vi "Processing_data_subvi_V23.vi"() -> ()   [LabVIEW 2025]
uses:
  <vilib>/Analysis/3filter.llb/Filter Passband Type.ctl
  <vilib>/Analysis/baseanly.llb/Mean (DBL).vi
  <vilib>/Utility/file.llb/Read Delimited Spreadsheet (DBL).vi
  <vilib>/Analysis/1siggen.llb/Ramp Pattern by Delta.vi
  <vilib>/Analysis/3filter.llb/Butterworth Filter (DBL).vi
  <vilib>/addons/Time Series Analysis/Series Preprocess.llb/TSA Moving Average (Array).vi
  <vilib>/addons/Time Series Analysis/Correlation and Spectral Analysis.llb/TSA AR Spectrum (Array).vi
  <vilib>/Analysis/NI_AAL_SigProc.lvlib
  <vilib>/Analysis/NI_AALBase.lvlib
  <vilib>/Analysis/NI_AALPro.lvlib
  <vilib>/addons/_Advanced Signal Processing/NI_AdvSigProcTSA.lvlib
panel:
  in  "Path":path
  out "TABLE:TIME DOMAIN ANALYSES":string[][](table)
  in  "Sampling Frecuency [Hz]":dbl=500.0 format="%#_13g"
  out "ECG adquired":cluster{dbl[], "all rows":dbl[]}(graph)
  out "Tachograme":dbl[](graph)
  out "HF power_n":dbl
  out "LF power_n":dbl
  out "VLF Power [ms²]":dbl
  out "Ratio LF/HF":dbl
  out "HF power [ms²]":dbl
  out "LF power [ms²]":dbl
  out "AR methode":cluster{dbl[], dbl[]}[](graph)
  out "Mean Heart Rate [bpm]":dbl
  out "pRR50 %":dbl
  out "RMSS":dbl
  out "Min RR interval [ms]":dbl
  out "Max RR interval [ms]":dbl
  out "Std RR interval  [ms]":dbl format="%0.2f"
  out "Mean RR interval [ms]":dbl format="%0.2f"
  out "MWI":dbl[](graph)
  out "Squared signal":dbl[](graph)
  out "Derivated signal":dbl[](graph)
  out "Filter ECG":dbl[](graph)
  out "HRV mean":dbl format="%0.2f"
  out "HRV (ms)":dbl[](array[numeric])
  in  "file path (use dialog)":path
  out "Intervals R-R":dbl[](array[numeric])
  # "TIME DOMAIN ANALYSES"
  # "HEART RATE VARIABILITY ESTIMATORS FOR STRESS DETECTION"
  # "MARCON Pietro, MAZZANTE Lorenzo, SCORZA Martín"
  # "FRECUENCY DOMAIN ANALYSES"
  # "BM04 -Université de technologie de Compiègne"
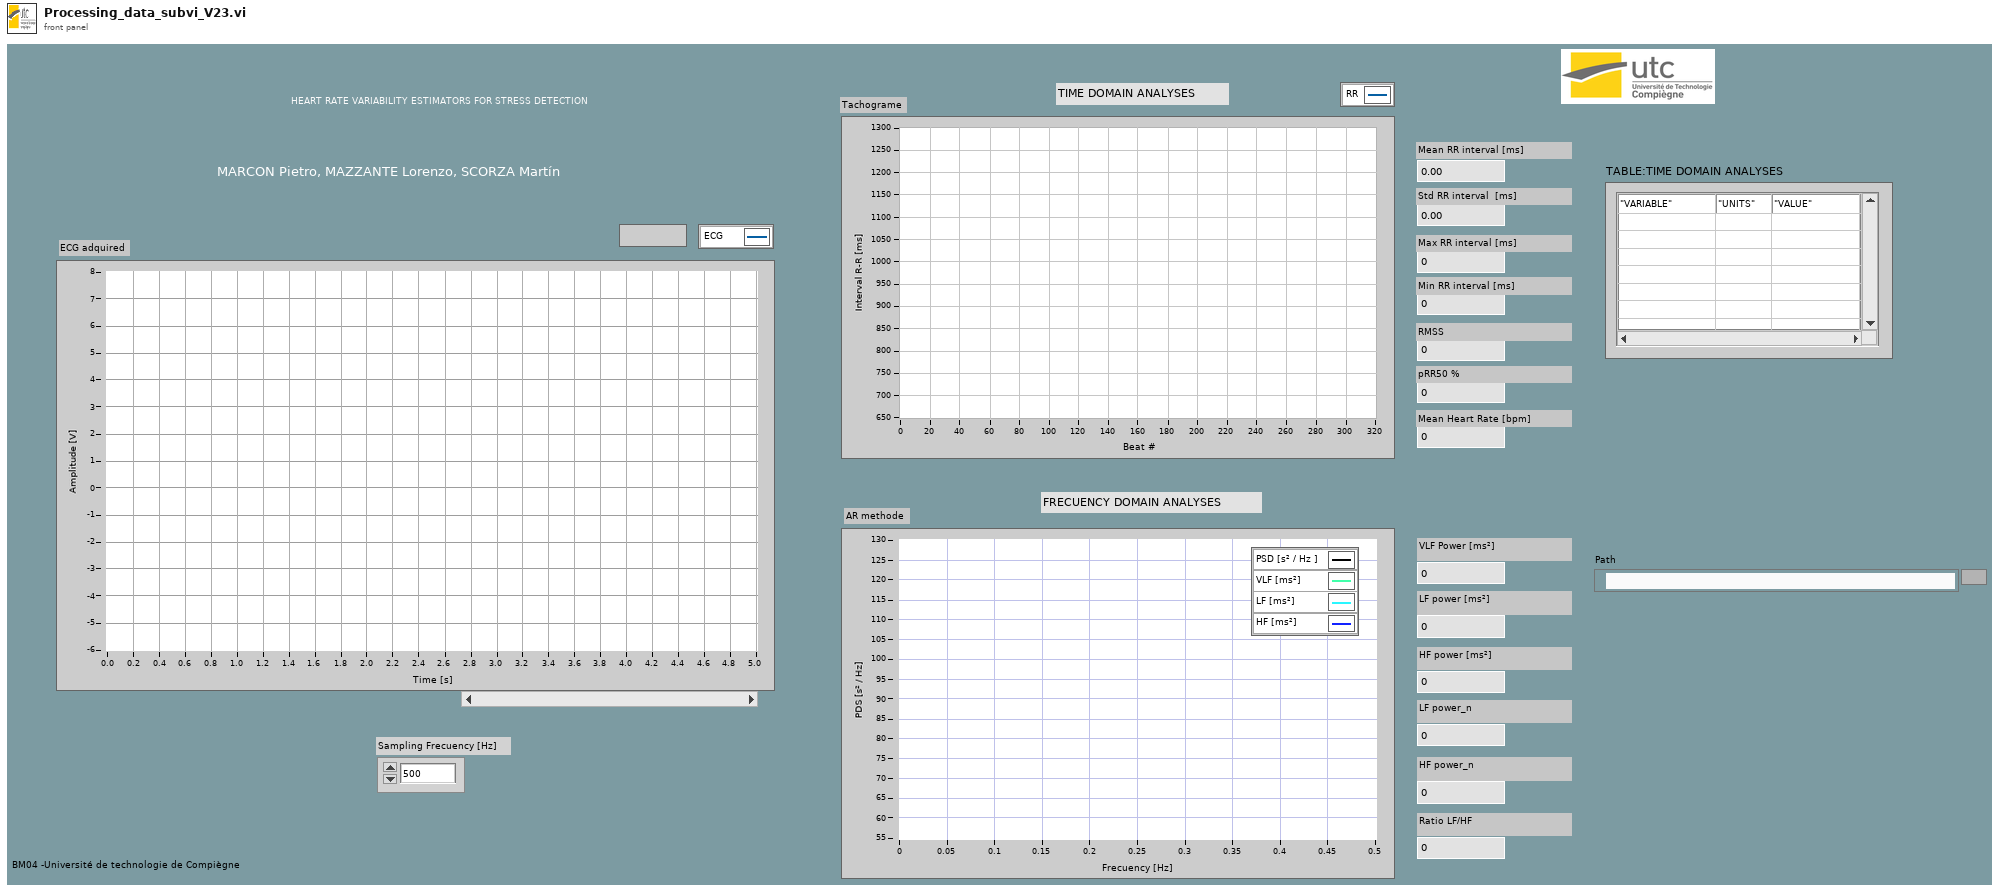
[diagram p1: front panel]
types:
  T1 = typedef "NI_AALBase.lvlib/Filter Passband Type.ctl" = enum32{"Lowpass", "Highpass", "Bandpass", "Bandstop"}
  T2 = cluster{cluster{dbl[], dbl[]}, cluster{dbl[], dbl[]}, cluster{dbl[], dbl[]}, cluster{dbl[], dbl[]}}
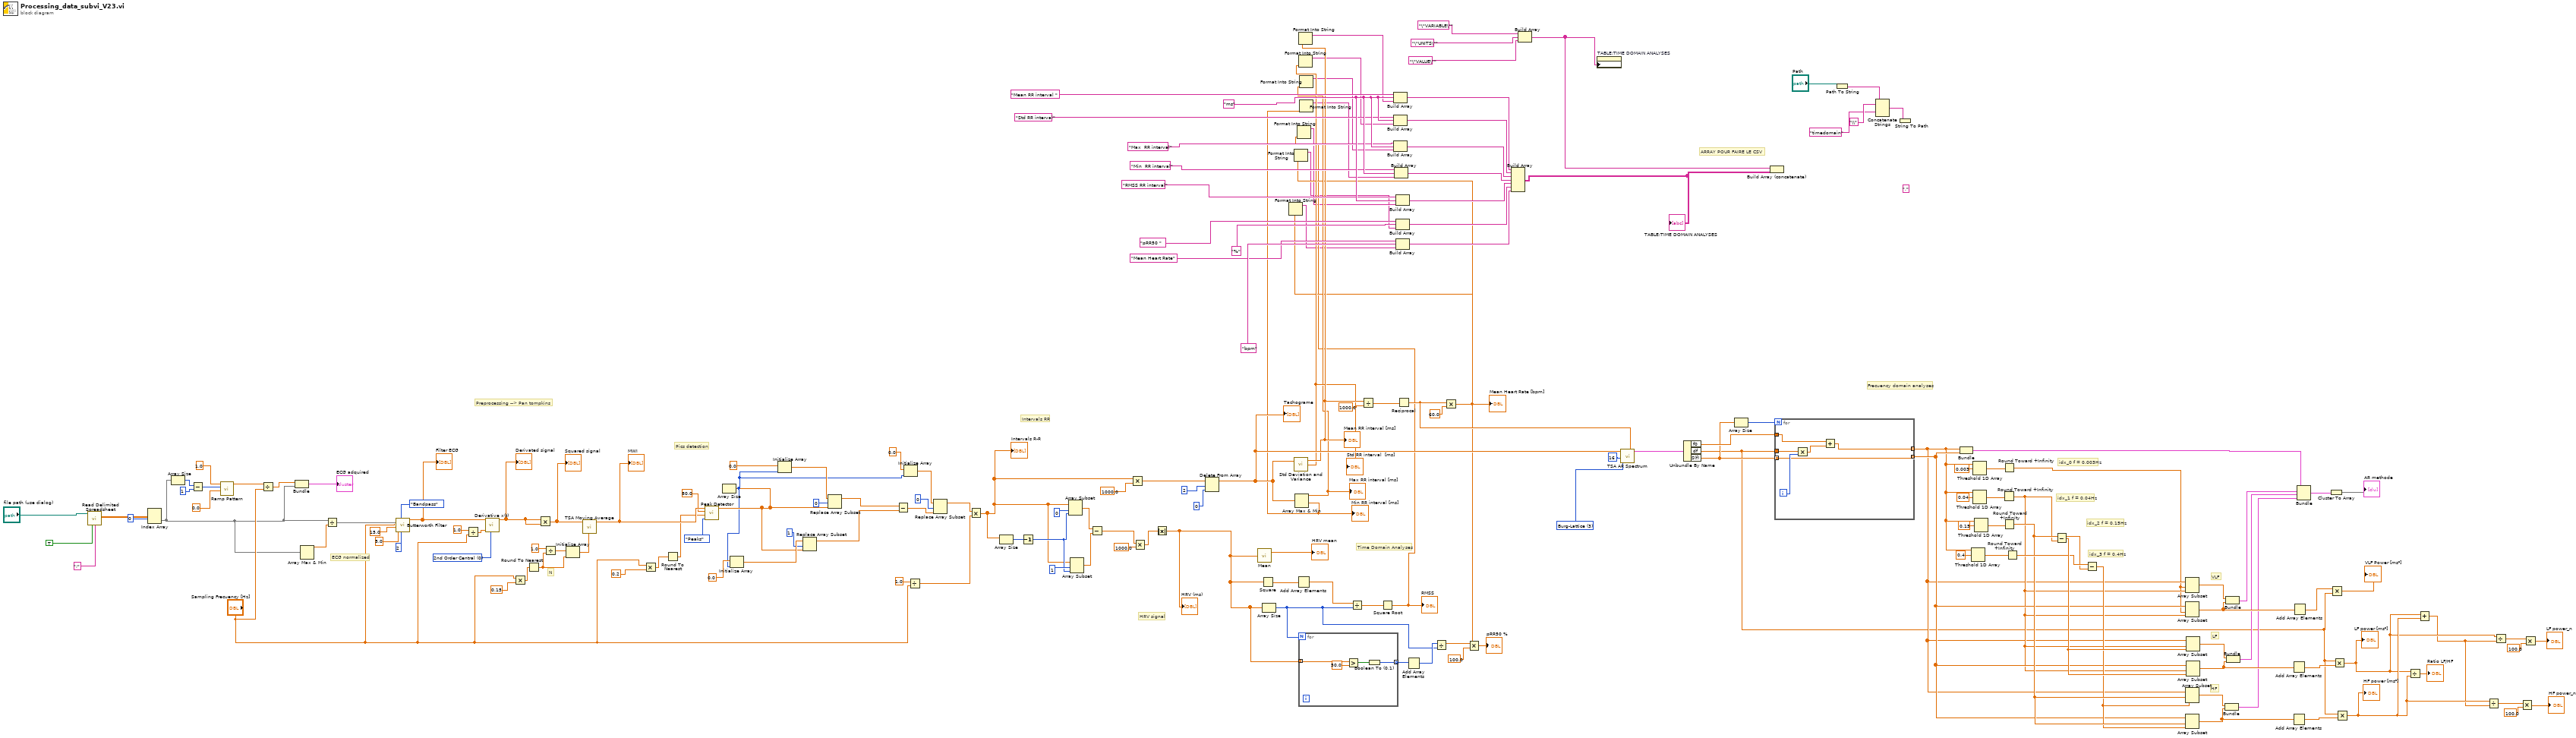
[diagram p0: block diagram]
diagram:
  w7 = "," ("delimiter (\\t)")
  w43 = "ms"
  w118 = u16 3 items=["Forward-Backward", "Least-Squares", "Yule-Walker", "Burg-Lattice", "Geometric-Lattice"] ("AR method")
  w141 = u16 0 items=["2nd Order Central", "4th Order Central", "Forward", "Backward"] ("method")
  # "ARRAY POUR FAIRE LE CSV"
  # "Frecuency domain analyses"
  # "ECG normalized"
  # "idx_0 f = 0,003Hz"
  # "VLF"
  # "HF"
  # "LF"
  # "idx_3 f = 0,4Hz"
  # "idx_2 f = 0,15Hz"
  # "idx_1 f = 0,04Hz"
  # "HRV signal"
  # "Intervals RR"
  # "Pics detection"
  # "Time Domain Analyses"
  # "Preprocessing --> Pan tompkins"
  # "N"
  n1 = call-poly <vilib>:"Read Delimited Spreadsheet.vi"("file path (dialog if empty)"="file path (use dialog)", "transpose? (F)"=TRUE, "delimiter (\\t)"=";" ("delimiter (\\t)")) -> ("all rows"=w161:dbl[][])  [unwired: 7 in, 5 out]
  n2 = Index Array(array=w161, index (row)=0) -> (element=w53:dbl[])  [unwired: 1 in]
  n3 = Array Size(array=w53) -> (size(s)=w59:i32)
  n4 = Subtract(x=w59, y=1) -> (x-y=w57:i32)
  n5 = call-poly <vilib>:"Ramp Pattern.vi"("start"=0.0, "end"=w57, "delta"=1.0) -> ("Ramp Pattern"=w55:dbl[])  [unwired: 6 in, 2 out]
  n6 = Divide(x=w55, y="Sampling Frecuency [Hz]") -> (x/y=w54:dbl[])
  n7 = Bundle(w54, "all rows"=w53) -> (→"ECG adquired":cluster{dbl[], "all rows":dbl[]})  [unwired: 1 in]
  n8 = Array Max & Min(array=w53) -> (max value=w66:dbl)  [unwired: 3 out]
  n9 = Divide(x=w53, y=w66) -> (x/y=w65:dbl[])
  n10 = call-poly <vilib>:"Butterworth Filter.vi"("order"=2, "filter type"=Filter_Passband_Type."Bandpass", "low cutoff freq: fl"=5.0, "high cutoff freq: fh"=15.0, "sampling freq: fs"="Sampling Frecuency [Hz]", "X"=w65) -> ("Filtered X"=w144:dbl[])  [unwired: 2 in, 1 out]
  "Filter ECG" <- w144
  n11 = Divide(x=1.0, y="Sampling Frecuency [Hz]") -> (x/y=w142:dbl)
  n12 = call <vilib>:"Derivative x(t).vi"("method"=w141, "dt"=w142, "X"=w144) -> ("dX/dt"=w140:dbl[])  [unwired: 7 in, 1 out]
  "Derivated signal" <- w140
  n13 = Multiply(x="Sampling Frecuency [Hz]", y=0.15) -> (x*y=w134:dbl)
  n14 = Round To Nearest(number=w134) -> (nearest integer value=w138:dbl)
  n15 = Multiply(x=w140, y=w140) -> (x*y=w62:dbl[])
  "Squared signal" <- w62
  n16 = Divide(x=1.0, y=w138) -> (x/y=w139:dbl)
  n17 = Initialize Array(w139, w138) -> (w136:dbl[])
  n18 = call-poly <vilib>:"TSA Moving Average.vi"("user defined weights"=w136, "Xt"=w62) -> ("Xt out"=w133:dbl[])  [unwired: 8 in, 1 out]
  "MWI" <- w133
  n19 = Multiply(x="Sampling Frecuency [Hz]", y=0.2) -> (x*y=w130:dbl)
  n20 = Round To Nearest(number=w130) -> (nearest integer value=w129:dbl)
  n21 = call <vilib>:"Peak Detector.vi"("peaks/valleys"=enum32{"Peaks", "Valleys"}."Peaks", "width"=w129, "threshold"=80.0, "X"=w133) -> ("Locations"=w173:dbl[])  [unwired: 3 in, 4 out]
  n22 = Array Size(array=w173) -> (size(s)=w170:i32)
  n23 = Initialize Array(0.0 ("element"), w170) -> (w174:dbl[])
  n24 = Initialize Array(0.0 ("element"), w170) -> (w177:dbl[])
  n25 = Replace Array Subset(array=w174, new element=w173, index=1) -> (w168:dbl[])
  n26 = Replace Array Subset(array=w177, new element=w173, index=0) -> (w169:dbl[])
  n27 = Subtract(x=w169, y=w168) -> (x-y=w166:dbl[])
  n28 = Initialize Array(0.0 ("element"), w170) -> (w167:dbl[])
  n29 = Divide(x=1.0, y="Sampling Frecuency [Hz]") -> (x/y=w67:dbl)
  n30 = Replace Array Subset(array=w167, new element=w166, index=0) -> (w159:dbl[])
  n31 = Multiply(x=w159, y=w67) -> (x*y=w64:dbl[])
  "Intervals R-R" <- w64
  n32 = Array Size(array=w64) -> (size(s)=w158:i32)
  n33 = Decrement(x=w158) -> (x-1=w153:i32)
  n34 = Array Subset(array=w64, index=0, length=w153) -> (w157:dbl[])
  n35 = Array Subset(array=w64, index=1, length=w153) -> (w154:dbl[])
  n36 = Subtract(x=w157, y=w154) -> (x-y=w151:dbl[])
  n37 = Multiply(x=w64, y=1000.0) -> (x*y=w50:dbl[])
  n38 = Multiply(x=w151, y=1000.0) -> (x*y=w150:dbl[])
  n39 = Absolute Value(x=w150) -> (abs(x)=w117:dbl[])
  "HRV (ms)" <- w117
  n40 = Delete From Array(array=w50, length=2, index=0) -> (array with subset deleted=w49:dbl[])  [unwired: 1 out]
  "Tachograme" <- w49
  n41 = call-poly <vilib>:"Mean.vi"("X"=w117) -> ("mean"=→"HRV mean":dbl)  [unwired: 1 out]
  n42 = Square(x=w117) -> (x^2=w126:dbl[])
  n43 = Array Size(array=w117) -> (size(s)=w120:i32)
  n44 = call <vilib>:"Std Deviation and Variance.vi"("X"=w49) -> ("mean"=w27:dbl, "standard deviation"=w26:dbl)  [unwired: 1 in, 1 out]
  "Mean RR interval [ms]" <- w27
  "Std RR interval  [ms]" <- w26
  n45 = Array Max & Min(array=w49) -> (max value=w25:dbl, min value=w22:dbl)  [unwired: 2 out]
  "Max RR interval [ms]" <- w25
  "Min RR interval [ms]" <- w22
  n46 = Add Array Elements(numeric array=w126) -> (sum=w125:dbl)
  n47 = Format Into String(w27) -> (resulting string=w17:string)  [unwired: 3 in, 1 out]
  n48 = Format Into String(w26) -> (resulting string=w16:string)  [unwired: 3 in, 1 out]
  n49 = for {
    N: w120 -> [_]
    tunnel: w117 -> [w182] mode=indexing
    tunnel: [w179] -> w124 mode=indexing
    n50 = Greater?(x=w182, y=50.0) -> (0:w180:bool)
    n51 = Boolean To (0,1)(Boolean=w180) -> (0, 1=w179:i16)
  }
  n52 = Format Into String(w25) -> (resulting string=w15:string)  [unwired: 3 in, 1 out]
  n53 = Format Into String(w22) -> (resulting string=w14:string)  [unwired: 3 in, 1 out]
  n54 = Divide(x=w125, y=w120) -> (x/y=w127:dbl)
  n55 = Divide(x=w27, y=1000.0) -> (x/y=w113:dbl)
  n56 = Square Root(x=w127) -> (sqrt(x)=w21:dbl)
  "RMSS" <- w21
  n57 = Format Into String(w21) -> (resulting string=w13:string)  [unwired: 3 in, 1 out]
  n58 = Build Array("Mean RR interval ", w43, w17) -> (w34:string[])
  n59 = Build Array("Std RR interval", w43, w16) -> (w33:string[])
  n60 = Build Array("Max  RR interval", w43, w15) -> (w32:string[])
  n61 = Build Array("Min  RR interval", w43, w14) -> (w31:string[])
  n62 = Build Array("RMSS RR interval", w43, w13) -> (w30:string[])
  n63 = Reciprocal(x=w113) -> (1/x=w46:dbl)
  n64 = Add Array Elements(numeric array=w124) -> (sum=w123:i16)
  n65 = Divide(x=w123, y=w120) -> (x/y=w122:dbl)
  n66 = Multiply(x=w46, y=60.0) -> (x*y=w23:dbl)
  "Mean Heart Rate [bpm]" <- w23
  n67 = Format Into String(w23) -> (resulting string=w11:string)  [unwired: 3 in, 1 out]
  n68 = Build Array("Mean Heart Rate", "bpm", w11) -> (w28:string[])
  n69 = Multiply(x=w122, y=100.0) -> (x*y=w24:dbl)
  "pRR50 %" <- w24
  n70 = Format Into String(w24) -> (resulting string=w12:string)  [unwired: 3 in, 1 out]
  n71 = Build Array("pRR50 ", "%", w12) -> (w29:string[])
  n72 = Build Array(w34, w33, w32, w31, w30, w29, w28) -> (w9:string[][])
  "TABLE:TIME DOMAIN ANALYSES" <- w9
  n73 = Build Array("\"VARIABLE\"", "\"UNITS\"", "\"VALUE\"") -> (w10:string[])
  n74 = property on="TABLE:TIME DOMAIN ANALYSES" class="Tbl (strict)"("Column Headers[]"=w10) -> ()  [unwired: 2 in, 2 out]
  n75 = call-poly <vilib>:"TSA AR Spectrum.vi"("sampling rate"=w46, "AR order"=16, "AR method"=w118, "Xt"=w49) -> ("PSD"=w116:cluster{"f0":dbl, "df":dbl, "S(f)":dbl[]})  [unwired: 6 in, 1 out]
  n76 = Unbundle By Name(w116) -> ("f0"=w111:dbl, "df"=w63:dbl, "S(f)"=w110:dbl[])
  n77 = Array Size(array=w110) -> (size(s)=w112:i32)
  n78 = Build Array (concatenate)(w10, w9) -> (w8:string[][])
  n79 = for {
    N: w112 -> [_]
    tunnel: w111 -> [w185]
    tunnel: w63 -> [w188]
    tunnel: w110 -> [w186] mode=indexing
    tunnel: [w186] -> w88 mode=indexing
    tunnel: [w183] -> w69 mode=indexing
    i -> [w187]
    n80 = Multiply(x=w188, y=w187) -> (x*y=w184:dbl)
    n81 = Add(x=w185, y=w184) -> (x+y=w183:dbl)
  }
  n82 = Path To String(path="Path") -> (string=w5:string)
  n83 = Concatenate Strings(w5, "\\" ("string"), "timedomain" ("string")) -> (w3:string)  [unwired: 2 in]
  n84 = String To Path(string=w3) -> (path=w2:path)
  n85 = Bundle(w69, w88) -> (w97:cluster{dbl[], dbl[]})  [unwired: 1 in]
  n86 = Threshold 1D Array(2:0.4 ("threshold y"), 3:w69) -> (0:w104:dbl)  [unwired: 1 in]
  n87 = Threshold 1D Array(2:0.04 ("threshold y"), 3:w69) -> (0:w106:dbl)  [unwired: 1 in]
  n88 = Threshold 1D Array(2:0.003 ("threshold y"), 3:w69) -> (0:w70:dbl)  [unwired: 1 in]
  n89 = Threshold 1D Array(2:0.15 ("threshold y"), 3:w69) -> (0:w105:dbl)  [unwired: 1 in]
  n90 = Round Toward +Infinity(x=w106) -> (ceil(x): smallest int >= x=w87:dbl)
  n91 = Round Toward +Infinity(x=w70) -> (ceil(x): smallest int >= x=w68:dbl)
  n92 = Round Toward +Infinity(x=w105) -> (ceil(x): smallest int >= x=w101:dbl)
  n93 = Round Toward +Infinity(x=w104) -> (ceil(x): smallest int >= x=w102:dbl)
  n94 = Subtract(x=w101, y=w87) -> (x-y=w103:dbl)
  n95 = Subtract(x=w102, y=w101) -> (x-y=w100:dbl)
  n96 = Array Subset(array=w69, index=w68, length=w87) -> (w89:dbl[])
  n97 = Array Subset(array=w88, index=w68, length=w87) -> (w86:dbl[])
  n98 = Array Subset(array=w69, index=w101, length=w100) -> (w98:dbl[])
  n99 = Array Subset(array=w88, index=w101, length=w100) -> (w93:dbl[])
  n100 = Array Subset(array=w69, index=w87, length=w103) -> (w99:dbl[])
  n101 = Array Subset(array=w88, index=w87, length=w103) -> (w94:dbl[])
  n102 = Bundle(w98, w93) -> (w82:cluster{dbl[], dbl[]})  [unwired: 1 in]
  n103 = Bundle(w89, w86) -> (w84:cluster{dbl[], dbl[]})  [unwired: 1 in]
  n104 = Bundle(w99, w94) -> (w83:cluster{dbl[], dbl[]})  [unwired: 1 in]
  n105 = Add Array Elements(numeric array=w94) -> (sum=w92:dbl)
  n106 = Add Array Elements(numeric array=w93) -> (sum=w91:dbl)
  n107 = Add Array Elements(numeric array=w86) -> (sum=w85:dbl)
  n108 = Bundle(w97, w84, w83, w82) -> (w96:T2)  [unwired: 1 in]
  n109 = Cluster To Array(cluster=w96) -> (array=→"AR methode":cluster{dbl[], dbl[]}[])
  n110 = Multiply(x=w85, y=w63) -> (x*y=→"VLF Power [ms²]":dbl)
  n111 = Multiply(x=w63, y=w92) -> (x*y=w74:dbl)
  "LF power [ms²]" <- w74
  n112 = Multiply(x=w63, y=w91) -> (x*y=w81:dbl)
  "HF power [ms²]" <- w81
  n113 = Divide(x=w74, y=w81) -> (x/y=→"Ratio LF/HF":dbl)
  n114 = Add(x=w74, y=w81) -> (x+y=w72:dbl)
  n115 = Divide(x=w81, y=w72) -> (x/y=w76:dbl)
  n116 = Divide(x=w74, y=w72) -> (x/y=w79:dbl)
  n117 = Multiply(x=w76, y=100.0) -> (x*y=→"HF power_n":dbl)
  n118 = Multiply(x=w79, y=100.0) -> (x*y=→"LF power_n":dbl)
